vi "FromClusterToTagBusScript.vi"(5 "process":T2={"param?"=TRUE, "Parameter Data Interface VI (blank=tag bus to parameters.vi)"="", "Result Data Interface VI (blank=results to tag bus.vi)"="", "reverse param?"=FALSE, "Rev. Result Interface VI (blank=results from tag bus.vi)"="", "Rev. Parameter Interface VI (blank=tag bus from parameters.vi)"="", "result?"=TRUE, "reverse result?"=FALSE}, 7 "output":T3={"enable?"=TRUE, "Data Interface VI (blank=tag bus to outputs.vi)"="", "Reverse Interface VI (blank=tag bus from outputs.vi)"="", "reverse?"=FALSE}, 8 "error in":errorcluster, 10 "input":T1={"enable?"=TRUE, "Data Interface VI (blank=input to tag bus.vi)"="", "reverse?"=FALSE, "Reverse Interface VI (blank=input from tag bus.vi)"=""}) -> (0 "error out":errorcluster)   [LabVIEW 2013, in "data interface script.lvlib"]
doc: "THis Vi scripts the index cluster and the VI to convert from a cluster into Tagbus"
uses:
  data interface script.lvlib
  Controls/input script control.ctl
  Controls/output script control.ctl
  Controls/processing script control.ctl
  Controls/ControlsProperties.ctl
  <vilib>/Utility/miscctls.llb/LVPointTypeDef.ctl
  Controls/StateCluster.ctl
  Controls/initialized references.ctl
  Controls/interface VI type.ctl
panel:
  in  "Fixed-Channel Runtime Class Path":path
  in  "Fixed-Channel Configuration Class Path":path
  # "Use this tool to update your Fixed-Channel Tag Bus Module any time you modify any of it's Input, Processing, Results, or Output clusters of channel data.  A modification includes adding or removing channels, changing a channel name, or changing a data type.\n\nSpecify the path of both the runtime and configuration classes of your Fixed-Channel TBM and run the VI to create updated versions"
  # "These settings are optional and only need to be specified before running this VI if you changed the name of your Data Interface VIs.\nEnabling a given boolean indicates you wish to script a function for that operation. \"Reverse\" operations are quite literally the opposite of normal operations. For example if \"output\" would normally require conversion from the tag bus into custom data, \"reverse\" would provide the interface for generating a tag bus from custom data. This can be useful for debugging."
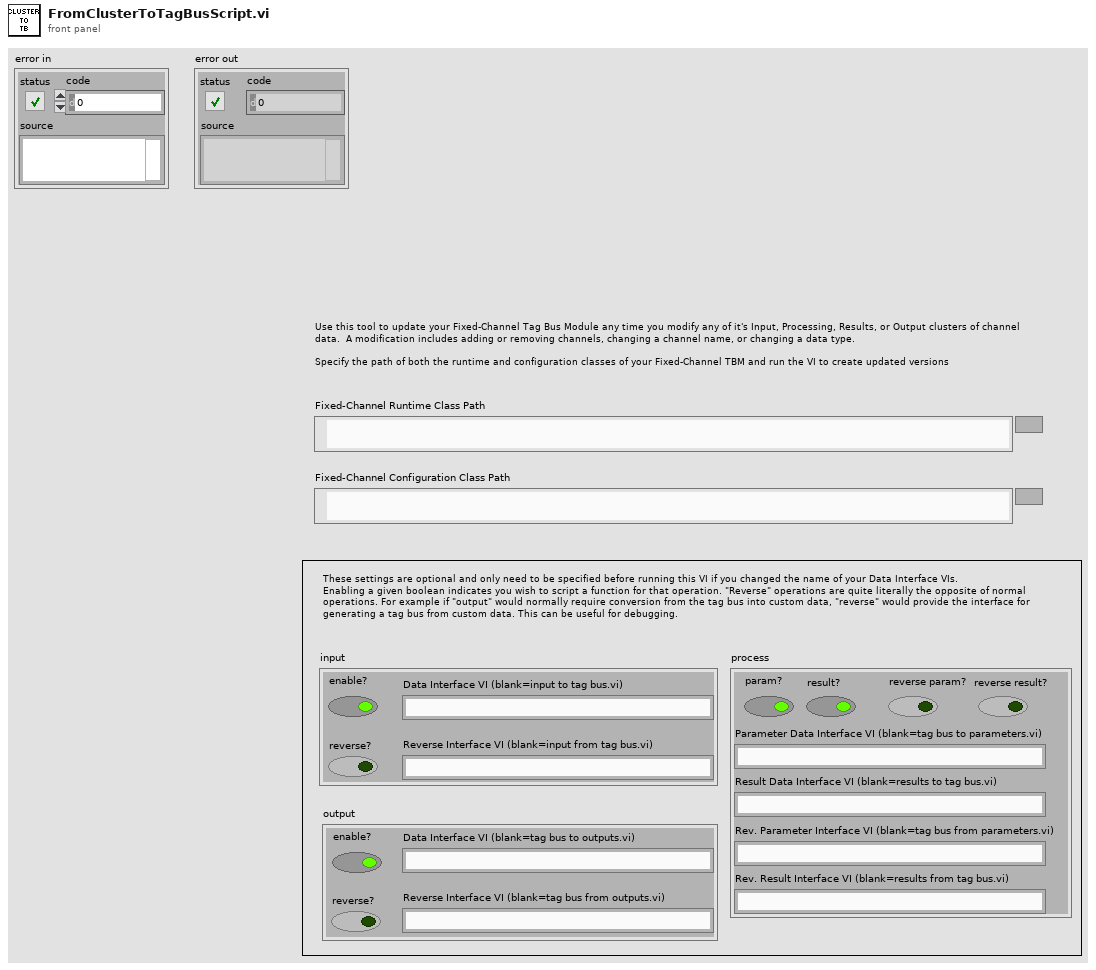
[diagram p1: front panel]
types:
  T1 = typedef "data interface script.lvlib/input script control.ctl" = cluster{"enable?":bool, "Data Interface VI (blank=input to tag bus.vi)":string, "reverse?":bool, "Reverse Interface VI (blank=input from tag bus.vi)":string}
  T2 = typedef "data interface script.lvlib/processing script control.ctl" = cluster{"param?":bool, "Parameter Data Interface VI (blank=tag bus to parameters.vi)":string, "Result Data Interface VI (blank=results to tag bus.vi)":string, "reverse param?":bool, "Rev. Result Interface VI (blank=results from tag bus.vi)":string, "Rev. Parameter Interface VI (blank=tag bus from parameters.vi)":string, "result?":bool, "reverse result?":bool}
  T3 = typedef "data interface script.lvlib/output script control.ctl" = cluster{"enable?":bool, "Data Interface VI (blank=tag bus to outputs.vi)":string, "Reverse Interface VI (blank=tag bus from outputs.vi)":string, "reverse?":bool}
  T4 = typedef "data interface script.lvlib/ControlsProperties.ctl" = cluster{"label":string, "terminal index":u32, "indicator":bool, "location":T5}
  T5 = typedef "LVPointTypeDef.ctl" = cluster{"Horizontal":i16, "Vertical":i16}
  T6 = typedef "data interface script.lvlib/initialized references.ctl" = cluster{"data ctl":refnum<vi>, "index ctl":refnum<vi>, "interface vi":refnum<vi>, "vi type":T7}
  T7 = typedef "data interface script.lvlib/interface VI type.ctl" = enum16{"tb to data", "data to tb"}
  T8 = typedef "data interface script.lvlib/StateCluster.ctl" = cluster{"base cluster":variant, "vi refs":T6}
  T9 = typedef "data interface script.lvlib/TerminalReferences.ctl" = cluster{"Cluster":refnum<vi>, "Index Cluster":refnum<vi>, "tag bus in":refnum<vi>, "tag bus out":refnum<vi>}
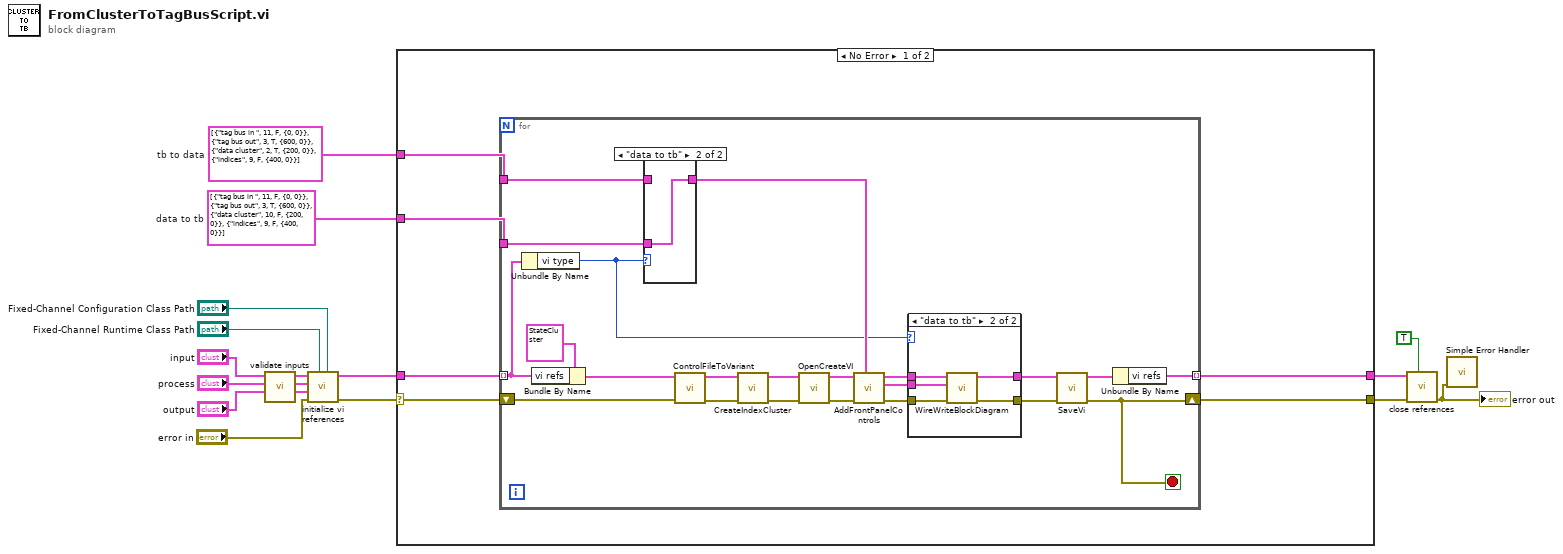
[diagram p0: block diagram]
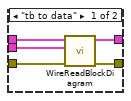
[diagram p2: hidden frame]
diagram:
  w4 = T4[] [{"label"="tag bus in ", "terminal index"=11, "indicator"=FALSE, "location"={"Horizontal"=0, "Vertical"=0}}, {"label"="tag bus out", "terminal index"=3, "indicator"=TRUE, "location"={"Horizontal"=600, "Vertical"=0}}, {"label"="data cluster", "terminal index"=10, "indicator"=FALSE, "location"={"Horizontal"=200, "Vertical"=0}}, {"label"="indices", "terminal index"=9, "indicator"=FALSE, "location"={"Horizontal"=400, "Vertical"=0}}]  # data to tb
  w5 = T4[] [{"label"="tag bus in ", "terminal index"=11, "indicator"=FALSE, "location"={"Horizontal"=0, "Vertical"=0}}, {"label"="tag bus out", "terminal index"=3, "indicator"=TRUE, "location"={"Horizontal"=600, "Vertical"=0}}, {"label"="data cluster", "terminal index"=2, "indicator"=TRUE, "location"={"Horizontal"=200, "Vertical"=0}}, {"label"="indices", "terminal index"=9, "indicator"=FALSE, "location"={"Horizontal"=400, "Vertical"=0}}]  # tb to data
  n1 = call "validate inputs.vi"("output in"="output", "process in"="process", "input in"="input") -> ("output out"=w12:T3, "process out"=w13:T2, "input out"=w14:T1)  [unwired: 6 in]
  n2 = call "initialize vi references.vi"("config class path"="Fixed-Channel Configuration Class Path", "runtime class path"="Fixed-Channel Runtime Class Path", "error in"="error in", "output in"=w12, "process in"=w13, "input in"=w14) -> ("error out"=w10:errorcluster, "initialized references"=w9:T6[])  [unwired: 4 in]
  n3 = case shown="No Error" w10 {
    selector: w10 -> [w22 w59]
    tunnel: w9 -> [w23 w58]
    tunnel: [w21 w59] -> w6
    tunnel: [w18 w58] -> w7
    tunnel: w5 -> [w20 _]
    tunnel: w4 -> [w19 _]
    frame No Error {
      n4 = for {
        tunnel: w23 -> [w42] mode=indexing
        shift-right: [w26] -> w21
        shift-left: w22 -> [w24]
        tunnel: w20 -> [w45]
        tunnel: w19 -> [w44]
        tunnel: [w27] -> w18 mode=indexing
        stop <- w26 stop-if-true
        n5 = Unbundle By Name(w42) -> ("vi type"=w34:T7)
        n6 = Bundle By Name(cluster=T8 {"base cluster"=variant, "vi refs"={"data ctl"=refnum, "index ctl"=refnum, "interface vi"=refnum, "vi type"=enum."tb to data"}} ("State"), "vi refs"=w42) -> (w25:T8)
        n7 = case shown="\"data to tb\"" w34 {
          tunnel: [w56 w57] -> w35
          tunnel: w45 -> [w56 _]
          tunnel: w44 -> [_ w57]
          frame "tb to data" {
          }
          frame "data to tb" {
          }
        }
        n8 = call "ControlFileToVariant.vi"("error in"=w24, "State"=w25) -> ("error out"=w40:errorcluster, "State out"=w41:T8)  [unwired: 8 in]
        n9 = call "CreateIndexCluster.vi"("error in"=w40, "State"=w41) -> ("error out"=w38:errorcluster, "State out"=w39:T8)  [unwired: 8 in]
        n10 = call "OpenCreateVI.vi"("error in"=w38, "State"=w39) -> ("error out"=w37:errorcluster, "State out"=w36:T8)  [unwired: 8 in]
        n11 = call "AddFrontPanelControls.vi"("Control Properties"=w35, "error in"=w37, "State"=w36) -> ("error out"=w31:errorcluster, "Terminal References"=w32:T9, "State out"=w33:T8)  [unwired: 6 in]
        n12 = case shown="\"data to tb\"" w34 {
          tunnel: w33 -> [w50 w55]
          tunnel: w32 -> [w49 w54]
          tunnel: w31 -> [w48 w53]
          tunnel: [w47 w52] -> w29
          tunnel: [w46 w51] -> w30
          frame "tb to data" {
            n13 = call "WireReadBlockDiagram.vi"("error in"=w48, "Terminal References"=w49, "State"=w50) -> ("error out"=w47:errorcluster, "State out"=w46:T8)  [unwired: 7 in]
          }
          frame "data to tb" {
            n14 = call "WireWriteBlockDiagram.vi"("error in"=w53, "Terminal References"=w54, "State"=w55) -> ("error out"=w52:errorcluster, "State out"=w51:T8)  [unwired: 7 in]
          }
        }
        n15 = call "SaveVi.vi"("error in"=w29, "State"=w30) -> ("error out"=w26:errorcluster, "State out"=w28:T8)  [unwired: 8 in]
        n16 = Unbundle By Name(w28) -> ("vi refs"=w27:T6)
      }
    }
    frame Error {
    }
  }
  n17 = call "close references.vi"("Open Front Panel"=TRUE, "error in"=w6, "initialized references"=w7) -> ("error out"=w1:errorcluster)  [unwired: 8 in]
  "error out" <- w1
  n18 = call <vilib>:"Simple Error Handler.vi"("error in (no error)"=w1) -> ()  [unwired: 4 in, 5 out]
